vi "8bit Cam Brightness and contrast.vi"(8 "error in (no error)":errorcluster, 9 "Ctrl refs":T1, 11 "8bit Input image":T2) -> (0 "error out":errorcluster, 3 "8bit Output image":T2)   [LabVIEW 2020]
uses:
  <vilib>/vision/Image Controls.llb/IMAQ Image.ctl
  Timelapse Viewer/Typedefs/8-bit video export window ctrl refs.ctl
  Typedefs/Bright-Contr-Gamma cluster.ctl
  Timelapse Viewer/Typedefs/Speed graph behaviour enum.ctl
  <vilib>/vision/NI_Vision_Development_Module.lvlib
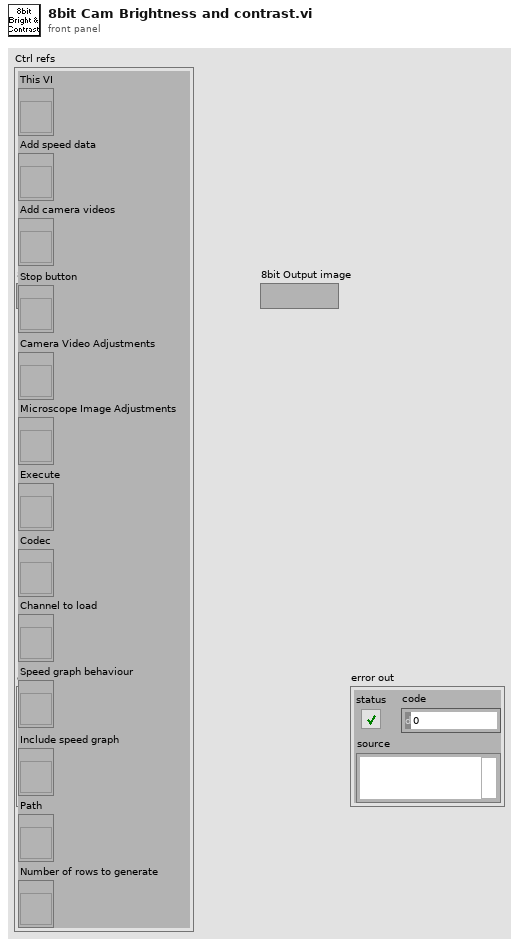
[diagram p1: front panel]
types:
  T1 = typedef "8-bit video export window ctrl refs.ctl" = cluster{"This VI":refnum<vi>, "Add speed data":refnum<vi>, "Add camera videos":refnum<vi>, "Stop button":refnum<vi>, "Camera Video Adjustments":refnum<vi>, "Microscope Image Adjustments":refnum<vi>, "Execute":refnum<vi>, "Codec":refnum<vi>, "Channel to load":refnum<vi>, "Speed graph behaviour":refnum<vi>, "Include speed graph":refnum<vi>, "Number of rows to generate":refnum<vi>, "Path":refnum<vi>}
  T2 = typedef "IMAQ Image.ctl" = refnum<image>
  T3 = typedef "Bright-Contr-Gamma cluster.ctl" = cluster{"Brightness":sgl, "Contrast":sgl, "Gamma":sgl}
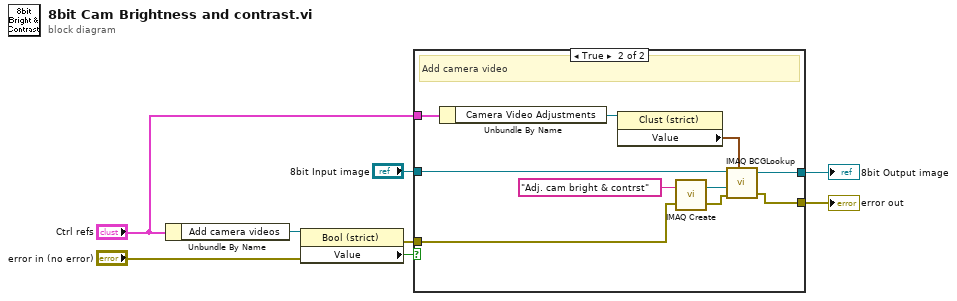
[diagram p0: block diagram]
diagram:
  n1 = Unbundle By Name("Ctrl refs") -> ("Add camera videos"=w8:refnum<vi>)
  n2 = property class="Bool (strict)"(reference=w8, error in="error in (no error)") -> (error out=w6:errorcluster, "Value"=w7:bool)  [unwired: 1 out]
  n3 = case shown="True" w7 {
    tunnel: [w9 w20] -> w3
    tunnel: [w10 w16] -> w4
    tunnel: w6 -> [w10 w15]
    tunnel: "8bit Input image" -> [w9 w19]
    tunnel: "Ctrl refs" -> [_ w13]
    frame False {
      # "Do not add camera video"
    }
    frame True {
      # "Add camera video"
      n4 = Unbundle By Name(w13) -> ("Camera Video Adjustments"=w12:refnum<vi>)
      n5 = property class="Clust (strict)"(reference=w12) -> ("Value"=w11:T3)  [unwired: 1 in, 2 out]
      n6 = call "IMAQ Create"("Image Name"="Adj. cam bright & contrst", "error in (no error)"=w15) -> ("New Image"=w17:T2, "error out"=w14:errorcluster)  [unwired: 3 in]
      n7 = call "IMAQ BCGLookup"("Image Src"=w19, "BCG Values"=w11, "Image Dst"=w17, "error in (no error)"=w14) -> ("Image Dst Out"=w20:T2, "error out"=w16:errorcluster)  [unwired: 3 in]
    }
  }
  "8bit Output image" <- w3
  "error out" <- w4
